vi "Save Accurate Data only.vi"(8 "error in":errorcluster, 10 "appended array":dbl[][](array[numeric]), 11 "configuration file path":path=path "C:/Users/User/Documents/setting.txt") -> (0 "error out 2":errorcluster, 3 "file path":path)   [LabVIEW 2023]
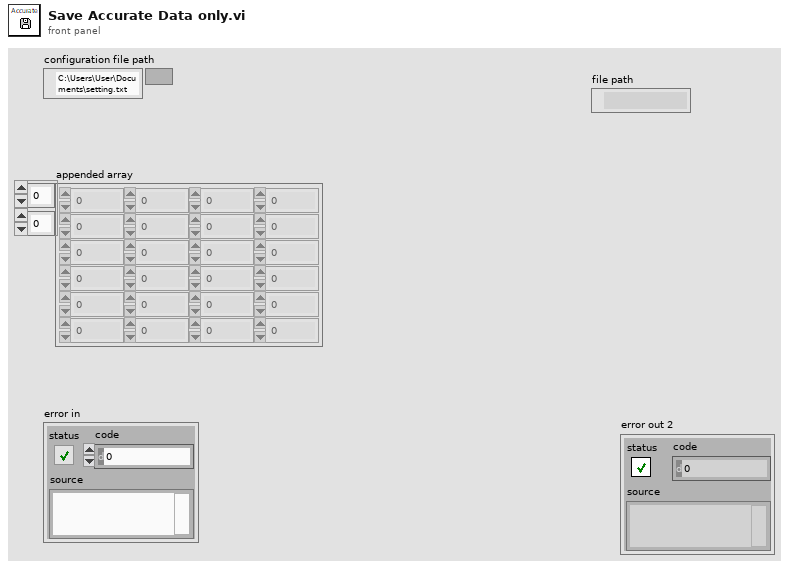
[diagram p1: front panel]
types:
  T1 = enum16{"open", "replace", "create", "open or create", "replace or create", "replace or create with confirmation"}
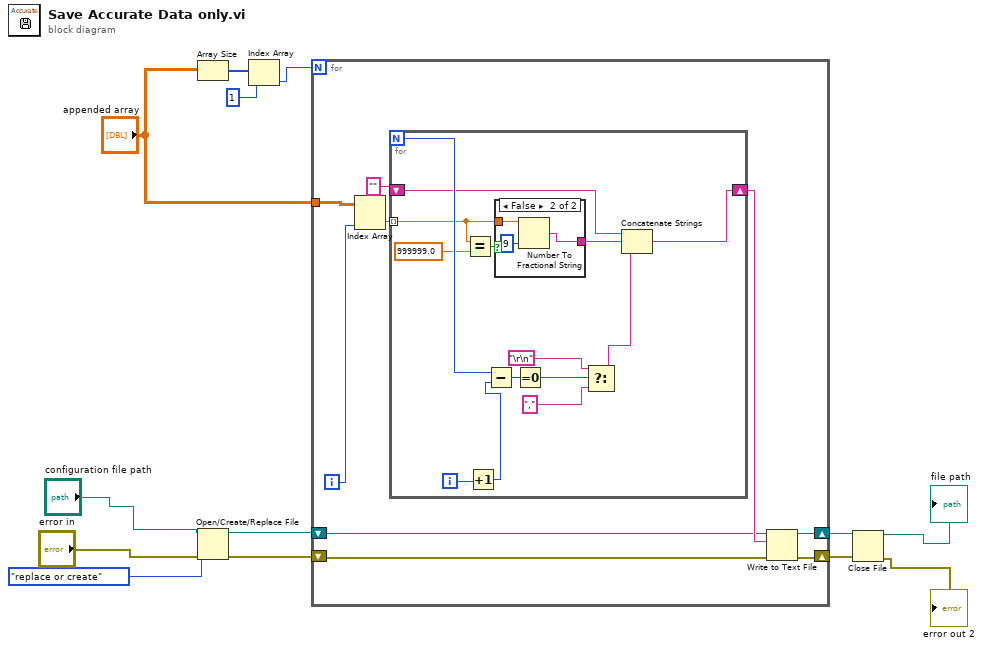
[diagram p0: block diagram]
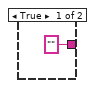
[diagram p2: hidden frame]
diagram:
  n1 = Array Size(array="appended array") -> (size(s)=w13:i32[])
  n2 = Open/Create/Replace File(file path (use dialog)="configuration file path", error in="error in", operation (0:open)=T1."replace or create") -> (refnum out=w7:refnum<file>, error out=w9:errorcluster)  [unwired: 3 in, 1 out]
  n3 = Index Array(array=w13, index=1) -> (element=w11:i32)
  n4 = for {
    N: w11 -> [_]
    tunnel: "appended array" -> [w22]
    shift-right: [w16] -> w8
    shift-left: w7 -> [w15]
    shift-right: [w14] -> w6
    shift-left: w9 -> [w18]
    i -> [w21]
    n5 = Index Array(array=w22, index (col)=w21) -> (element=w20:dbl[])  [unwired: 1 in]
    n6 = for {
      N -> [w32]
      tunnel: w20 -> [w24] mode=indexing
      shift-right: [w26] -> w17
      shift-left: "" -> [w27]
      i -> [w34]
      n7 = Equal?(x=w24, y=999999.0) -> (x = y?=w25:bool)
      n8 = Increment(x=w34) -> (x+1=w31:i32)
      n9 = Subtract(x=w32, y=w31) -> (x-y=w33:i32)
      n10 = case shown="False" w25 {
        tunnel: w24 -> [_ w40]
        tunnel: ["" w39] -> w36
        frame True {
        }
        frame False {
          n11 = Number To Fractional String(number=w40, precision (6)=i16 9) -> (F-format string=w39:string)  [unwired: 2 in]
        }
      }
      n12 = Equal To 0?(x=w33) -> (x = 0?=w35:bool)
      n13 = Select(t="\r\n", s=w35, f=",") -> (s? t:f=w28:string)
      n14 = Concatenate Strings(w27, w36, w28) -> (w26:string)
    }
    n15 = Write to Text File(file (use dialog)=w15, text=w17, error in=w18) -> (refnum out=w16:refnum<file>, error out=w14:errorcluster)  [unwired: 1 in, 1 out]
  }
  n16 = Close File(refnum=w8, error in=w6) -> (path=→"file path":path, error out=→"error out 2":errorcluster)
